vi "FRCts20_Backend_Revision_GET.vi"(8 "error in (no error)":errorcluster, 10 "Message Attributes":T4, 11 "Engine_Refnums":T1) -> (0 "error out":errorcluster)   [LabVIEW 2014, in "FRCts20_Backend_Engine.lvlib"]
uses:
  FRCts20_Backend_Engine.lvlib
  Dependencies/Keyed Array/KeyedArray.ctl
  FRCts20_Backend_EngineRefnums.ctl
  INI_Accessor/FRCts20_Backend_INI Controller.lvclass
  Dependencies/AMC/_SubVIs/TypeDefs/Message Queue.ctl
  Dependencies/AMC/_SubVIs/TypeDefs/Message.ctl
  <vilib>/addons/database/Connection.llb/Conn ObjectReference.ctl
  FRCts20_Backend_FGVOperation.ctl
  FRCts20_Backend_API/FRCts20_Backend_API_Application.ctl
  Dependencies/Keyed Array/Tools_KeyedArray.lvlib
  Dependencies/AMC/AMC.lvlib
  <vilib>/addons/database/NI_Database_API.lvlib
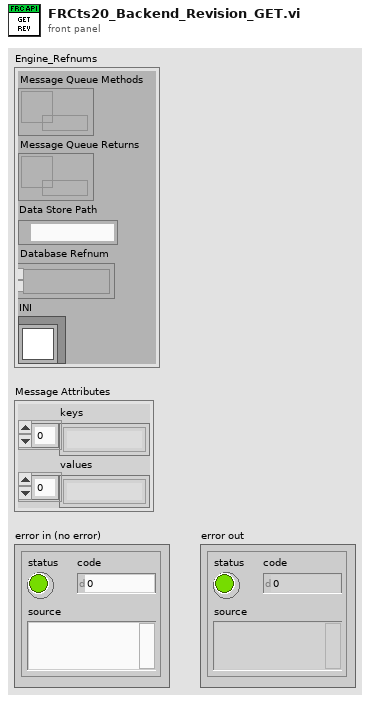
[diagram p1: front panel]
types:
  T1 = typedef "FRCts20_Backend_Engine.lvlib/FRCts20_Backend_EngineRefnums.ctl" = cluster{"Message Queue Methods":T2, "Message Queue Returns":T2, "Data Store Path":path, "Database Refnum":T3, "INI":refnum<class "FRCts20_Backend_INI Controller.lvclass">}
  T2 = typedef "AMC.lvlib/Message Queue.ctl" = refnum<queue>
  T3 = typedef "NI_Database_API.lvlib/Conn ObjectReference.ctl" = refnum<k1>
  T4 = typedef "Tools_KeyedArray.lvlib/KeyedArray.ctl" = cluster{"keys":string[], "values":string[]}
  T5 = typedef "FRCts20_Backend_API_Application.ctl" = cluster{"Revision":string, "APIReturn":string}
  T6 = typedef "FRCts20_Backend_Engine.lvlib/FRCts20_Backend_FGVOperation.ctl" = enum16{"Initialize", "EnqueueMessage", "EnqueueDataReturn", "FlushMessage", "FlushDataReturn"}
  T7 = typedef "FRCts20_Backend_Engine.lvlib/FRCts20_Backend_INI Controller.lvclass/FRCts20_Backend_INI_Revision.ctl" = cluster{"Major Revision":i32, "Minor Revision":i32, "Branch Number":i32, "Build Phase":string, "Build Number":i32}
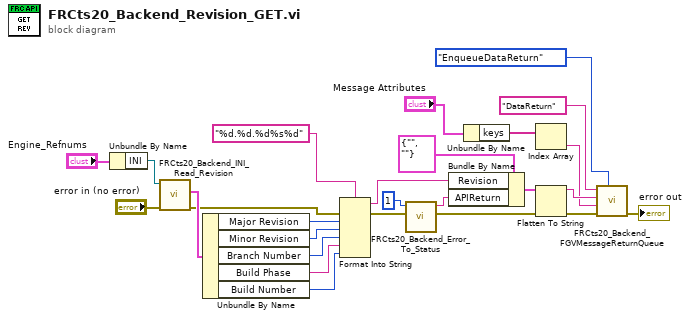
[diagram p0: block diagram]
diagram:
  n1 = Unbundle By Name("Engine_Refnums") -> ("INI"=w13:refnum<class "FRCts20_Backend_INI Controller.lvclass">)
  n2 = call "FRCts20_Backend_INI_Read_Revision.vi"("error in (no error)"="error in (no error)", "INI Controller in"=w13) -> ("error out"=w4:errorcluster, "Revision"=w6:T7)  [unwired: 7 in, 1 out]
  n3 = Unbundle By Name(w6) -> ("Major Revision"=w7:i32, "Minor Revision"=w8:i32, "Branch Number"=w9:i32, "Build Phase"=w11:string, "Build Number"=w10:i32)
  n4 = Format Into String(format string="%d.%d.%d%s%d", error in=w4, w7, w8, w9, w11, w10) -> (resulting string=w5:string, error out=w3:errorcluster)  [unwired: 1 in]
  n5 = call "FRCts20_Backend_Error_To_Status.vi"("error in (no error)"=w3, "rows affected"=1) -> ("error out"=w2:errorcluster, "String"=w1:string)  [unwired: 8 in]
  n6 = Bundle By Name(cluster=T5 {"Revision"="", "APIReturn"=""} ("Application"), "Revision"=w5, "APIReturn"=w1) -> (w25:T5)
  n7 = Unbundle By Name("Message Attributes") -> ("keys"=w20:string[])
  n8 = Index Array(array=w20) -> (element=w21:string)  [unwired: 1 in]
  n9 = Flatten To String(anything=w25, error in (no error)=w2) -> (data string=w24:string, error out=w23:errorcluster)  [unwired: 2 in, 1 out]
  n10 = call "FRCts20_Backend_FGVMessageReturnQueue.vi"("Operation"=FRCts20_Backend_FGVOperation."EnqueueDataReturn", "error in (no error)"=w23, "Key"=w21, "Message Value"=w24, "Message Name"="DataReturn") -> ("error out"=→"error out":errorcluster)  [unwired: 5 in, 1 out]
